vi "ActDriveStraightCalcError-ALT.vi"(10 "Dist (ft)":dbl, 11 "FirstTime":bool) -> (3 "Dist Error (Ft)":dbl)   [LabVIEW 2020]
uses:
  <vilib>/Rock Robotics/Network Tables/NT Write Number.vi
  <vilib>/Rock Robotics/Network Tables/NT Write Boolean.vi
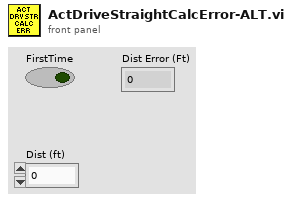
[diagram p1: front panel]
types:
  T1 = typedef "Trajectory_Library.lvlib/SWERVE_DRIVE_MODULE_POSITION.ctl" = cluster{"Distance":dbl, "Angle":T2, "P":bool}
  T2 = typedef "Trajectory_Library.lvlib/ROTATION2D.ctl" = cluster{"VALUE":dbl, "COS":dbl, "SIN":dbl}
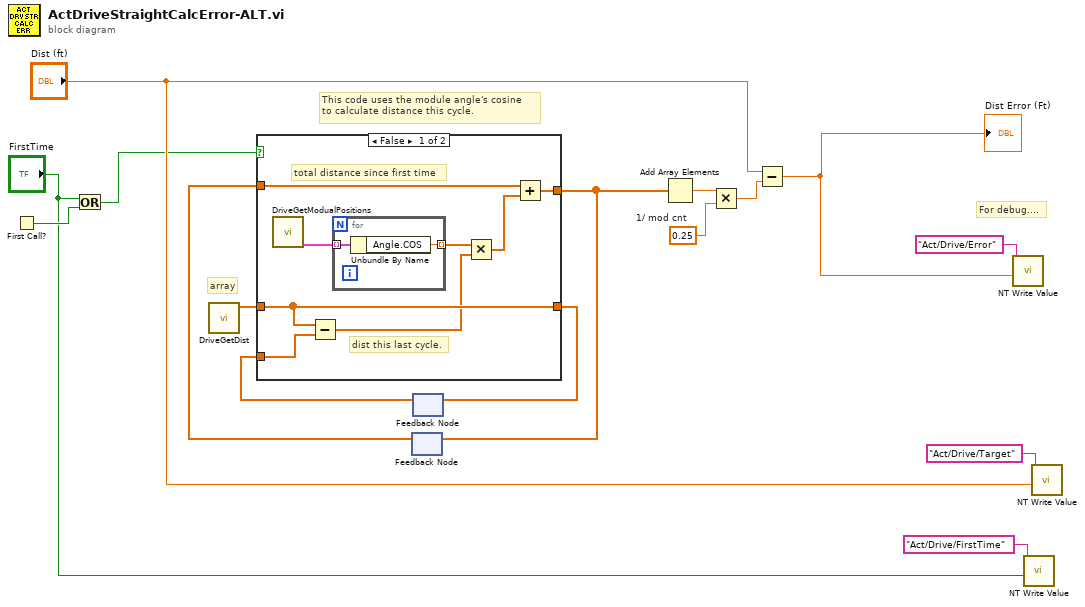
[diagram p0: block diagram]
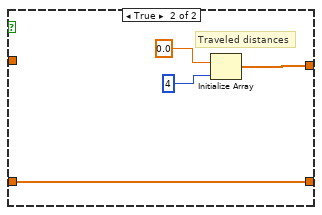
[diagram p2: hidden frame]
diagram:
  w13 = 0.25  # 1/ mod cnt
  # "For debug...."
  # "This code uses the module angle's cosine\nto calculate distance this cycle."
  # "array"
  n1 = First Call?() -> (First Call?: T/F=w3:bool)
  n2 = Or(x="FirstTime", y=w3) -> (x .or. y?=w2:bool)
  n3 = call "DriveGetDist.vi"() -> ("ModuleTravelPosition"=w9:dbl[])  [unwired: 11 in]
  n4 = feedback #1() -> (w14:dbl[])  [unwired: 1 in]
  n5 = feedback #2() -> (w15:dbl[])  [unwired: 1 in]
  n6 = case shown="False" w2 {
    tunnel: w9 -> [w21 w30]
    tunnel: [w21 w30] -> w16
    tunnel: [w23 w27] -> w11
    tunnel: w15 -> [w22 _]
    tunnel: w14 -> [w24 _]
    frame False {
      # "total distance since first time"
      # "dist this last cycle."
      n7 = call "DriveGetModualPositions.vi"() -> ("Swerve_Drive_Modual_Positions"=w17:T1[])  [unwired: 11 in]
      n8 = Subtract(x=w21, y=w22) -> (x-y=w19:dbl[])
      n9 = for {
        tunnel: w17 -> [w26] mode=indexing
        tunnel: [w25] -> w20 mode=indexing
        n10 = Unbundle By Name(w26) -> ("Angle.COS"=w25:dbl)
      }
      n11 = Multiply(x=w20, y=w19) -> (x*y=w18:dbl[])
      n12 = Add(x=w24, y=w18) -> (x+y=w23:dbl[])
    }
    frame True {
      # "Traveled distances"
      n13 = Initialize Array(0.0 ("element"), 4 ("dimension size")) -> (w27:dbl[])
    }
  }
  n14 = feedback-in #1(w11) -> ()
  n15 = feedback-in #2(w16) -> ()
  n16 = Add Array Elements(numeric array=w11) -> (sum=w12:dbl)
  n17 = Multiply(x=w12, y=w13) -> (x*y=w10:dbl)
  n18 = Subtract(x="Dist (ft)", y=w10) -> (x-y=w4:dbl)
  "Dist Error (Ft)" <- w4
  n19 = call-poly <vilib>:"NT Write Value.vi"("value"=w4, "name"="Act/Drive/Error") -> ()  [unwired: 9 in, 1 out]
  n20 = call-poly <vilib>:"NT Write Value.vi"("value"="FirstTime", "name"="Act/Drive/FirstTime") -> ()  [unwired: 9 in, 1 out]
  n21 = call-poly <vilib>:"NT Write Value.vi"("value"="Dist (ft)", "name"="Act/Drive/Target") -> ()  [unwired: 9 in, 1 out]
